vi "Write uStringManipulation.vi"(8 "error in (no error)":errorcluster, 10 "uStringManipulation.lvlibp:uStringManipulation.lvclass":refnum<class "uStringManipulation.lvclass">, 11 "uPolicy in":refnum<class "uPolicy.lvclass">) -> (0 "error out":errorcluster, 3 "uPolicy out":refnum<class "uPolicy.lvclass">)   [LabVIEW 2023, in "uFramework.lvlib" / "uPolicy.lvclass"]
uses:
  uPolicy.lvclass
  Bin/uStringManipulation.lvlibp/uStringManipulation.lvclass
  uPolicy.lvclass/uPolicy.ctl
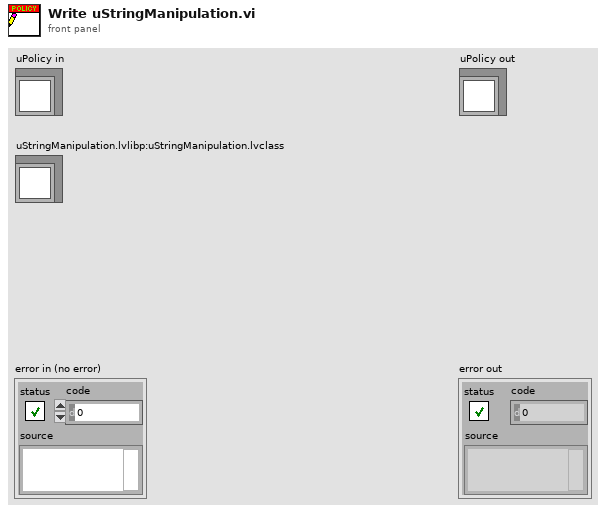
[diagram p1: front panel]
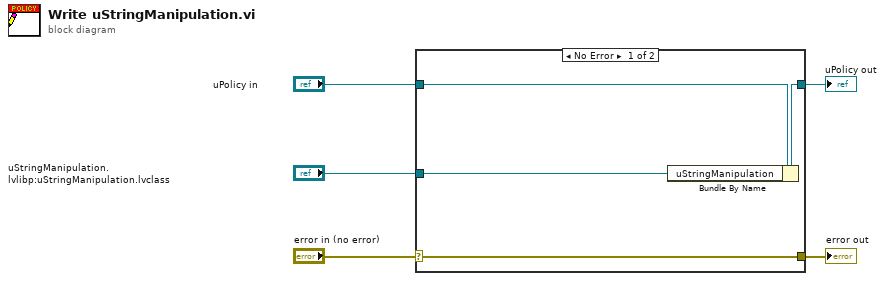
[diagram p0: block diagram]
diagram:
  n1 = case shown="No Error" "error in (no error)" {
    selector: "error in (no error)" -> [w9 w10]
    tunnel: [w9 w10] -> w4
    tunnel: [w7 w11] -> w2
    tunnel: "uPolicy in" -> [w8 w11]
    tunnel: "uStringManipulation.lvlibp:uStringManipulation.lvclass" -> [w6 _]
    frame No Error {
      n2 = Bundle By Name(cluster=w8, "uStringManipulation"=w6) -> (w7:refnum<class "uPolicy.lvclass">)
    }
    frame Error {
    }
  }
  "error out" <- w4
  "uPolicy out" <- w2
